vi "Init_E710_stage.vi"(4 "error in":errorcluster) -> (0 "error out":errorcluster, 3 "Stage Identification string":string)   [LabVIEW 2010, in "PI E710 Stage.lvlib"]
uses:
  PI E710 Stage.lvlib
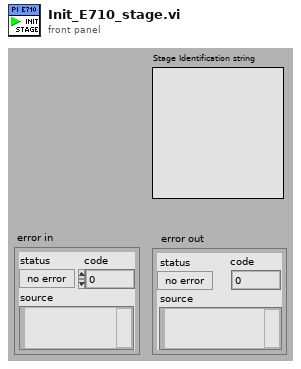
[diagram p1: front panel]
types:
  T1 = cluster{"input XON/XOFF":bool, "input HW Handshake":bool, "input alt HW HShk":bool, "output XON/XOFF":bool, "output HW Handshake":bool, "output alt HW HShk":bool, "XOFF byte ":u8, "XON byte":u8, "parity error byte":u16}
  T2 = cluster{"data bits":u16, "stop bits":enum16{"1 bit", "1.5 bits", "2 bits"}, "parity":enum16{"no parity", "odd parity", "even parity", "mark parity", "space parity"}}
  T3 = cluster{"RS232 Portnumber":u16, "Timeout":u32, "RS232 Baud rate":u32, "Interface":u16, "GPIB Bus":i32, "GPIB Address":i32, "GPIB Mode":i32}
  T4 = cluster{"DLL for Device":u16, "DLL Interface":u16, "Parameter":string}
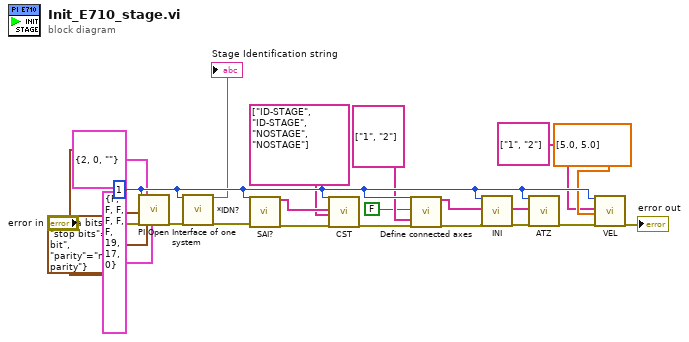
[diagram p0: block diagram]
diagram:
  w22 = 1 ("System\nnumber")
  n1 = call "PI Open Interface of one system.vi"("System\nnumber"=w22, "Interface configuration"=T3 {"RS232 Portnumber"=0, "Timeout"=5000, "RS232 Baud rate"=57600, "Interface"=2, "GPIB Bus"=0, "GPIB Address"=4, "GPIB Mode"=0}, "error in"="error in", "DLL Interface\nConfiguration"=T4 {"DLL for Device"=2, "DLL Interface"=0, "Parameter"=""} ("DLL Interface\nConfiguration"), "Bit settings and parity"=T2 {"data bits"=8, "stop bits"=enum."1 bit", "parity"=enum."no parity"}, "Flow control"=T1 {"input XON/XOFF"=FALSE, "input HW Handshake"=FALSE, "input alt HW HShk"=FALSE, "output XON/XOFF"=FALSE, "output HW Handshake"=FALSE, "output alt HW HShk"=FALSE, "XOFF byte "=19, "XON byte"=17, "parity error byte"=0}) -> ("error out"=w6:errorcluster)  [unwired: 13 in]
  n2 = call "*IDN?.vi"("System no."=w22, "error in"=w6) -> ("Identification"=→"Stage Identification string":string, "error out"=w9:errorcluster)  [unwired: 16 in]
  n3 = call "SAI?.vi"("System no."=w22, "error in"=w9) -> ("Conn. axes"=w12:string[], "error out"=w10:errorcluster)  [unwired: 16 in]
  n4 = call "CST.vi"("System no."=w22, "Axis ID's"=w12, "Stage names"=string[] ["ID-STAGE", "ID-STAGE", "NOSTAGE", "NOSTAGE"], "error in"=w10) -> ("error out"=w15:errorcluster)  [unwired: 15 in]
  n5 = call "Define connected axes.vi"("System no."=w22, "Read from\ncontroller?"=FALSE ("Read from\ncontroller?"), "Conn. axes"=string[] ["1", "2"], "error in"=w15) -> ("Conn. Axes out"=w18:string[], "error out"=w16:errorcluster)  [unwired: 14 in]
  n6 = call "INI.vi"("System no."=w22, "INI axes"=w18, "error in"=w16) -> ("error out"=w17:errorcluster)  [unwired: 16 in]
  n7 = call "ATZ.vi"("System no."=w22, "Affected axes"=w18, "error in"=w17) -> ("error out"=w19:errorcluster)  [unwired: 15 in, 1 out]
  n8 = call "VEL.vi"("System no."=w22, "Axes to set"=string[] ["1", "2"], "Velocity values"=dbl[] [5.0, 5.0], "error in"=w19) -> ("error out"=→"error out":errorcluster)  [unwired: 14 in, 1 out]
